vi "SquareFilter1.vi"(3 "error IN":errorcluster, 4 "Areas":dbl[][](array[numeric]), 5 "X,Y":dbl[][](array[numeric]), 6 "Chains (X,Y,dX,dY)":dbl[][](array[numeric])) -> (0 "error OUT":errorcluster, 1 "Finded False Displac":i32, 2 "Filtered Chains (X,Y,dX,dY)":dbl[][](array[numeric]))   [LabVIEW 2013]
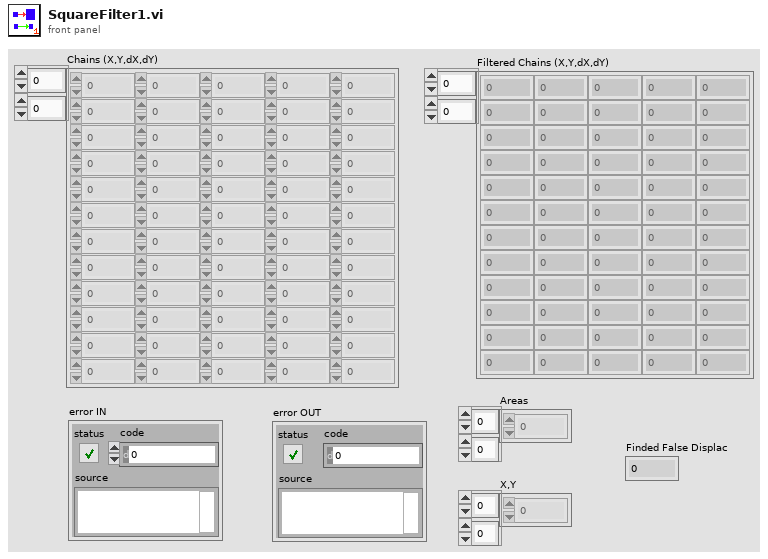
[diagram p1: front panel]
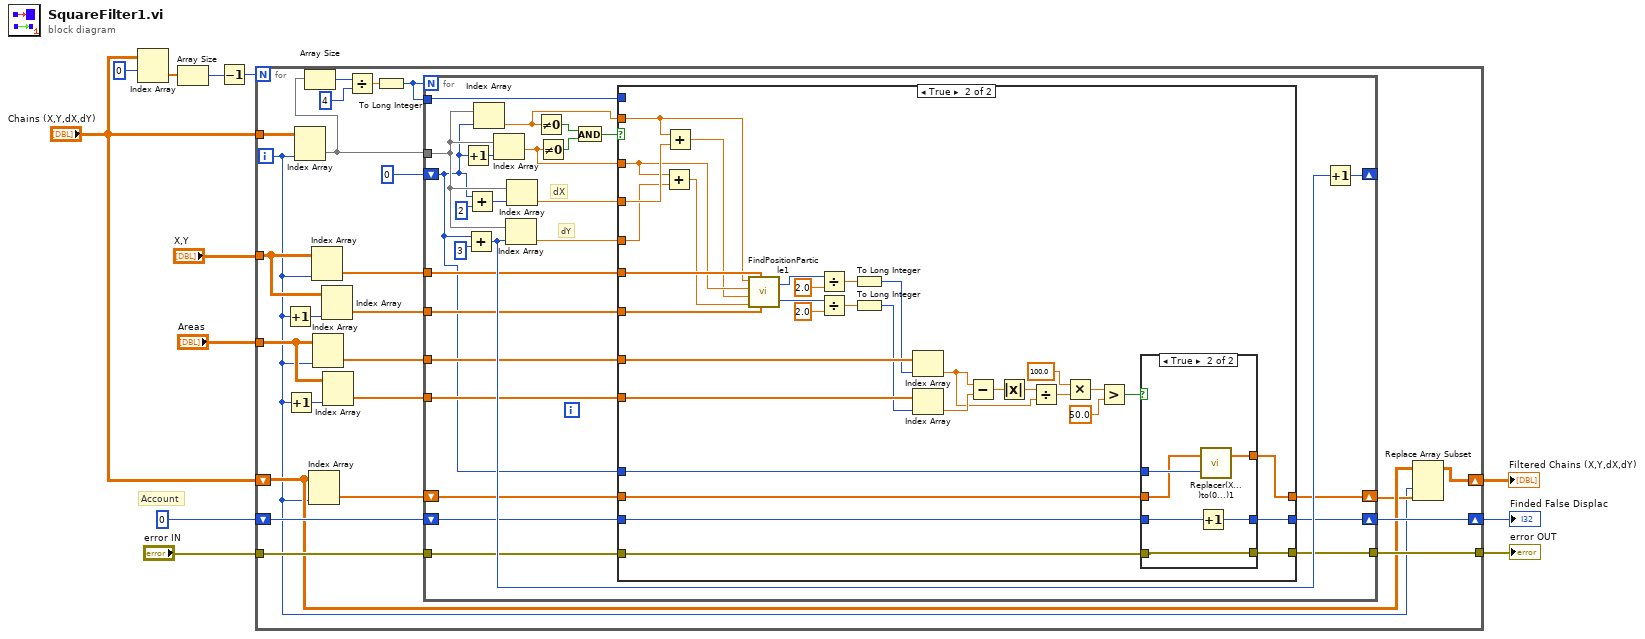
[diagram p0: block diagram]
diagram:
  # "Account"
  n1 = Index Array(array="Chains (X,Y,dX,dY)", index (row)=0) -> (element=w11:dbl[])  [unwired: 1 in]
  n2 = Array Size(array=w11) -> (size(s)=w4:i32)
  n3 = Decrement(x=w4) -> (x-1=w3:i32)
  n4 = for {
    N: w3 -> [_]
    tunnel: "error IN" -> [w33]
    tunnel: "Chains (X,Y,dX,dY)" -> [w31]
    shift-right: [w14] -> w6
    shift-left: "Chains (X,Y,dX,dY)" -> [w16]
    tunnel: [w30] -> w8
    shift-right: [w28] -> w7
    shift-left: 0 -> [w29]
    tunnel: "Areas" -> [w20]
    tunnel: "X,Y" -> [w25]
    i -> [w13]
    n5 = Increment(x=w13) -> (x+1=w24:i32)
    n6 = Increment(x=w13) -> (x+1=w21:i32)
    n7 = Index Array(array=w31, index (col)=w13) -> (element=w34:dbl[])  [unwired: 1 in]
    n8 = Array Size(array=w34) -> (size(s)=w36:i32)
    n9 = Index Array(array=w16, index (col)=w13) -> (element=w17:dbl[])  [unwired: 1 in]
    n10 = Index Array(array=w25, index (col)=w13) -> (element=w23:dbl[])  [unwired: 1 in]
    n11 = Index Array(array=w20, index (col)=w13) -> (element=w19:dbl[])  [unwired: 1 in]
    n12 = Index Array(array=w25, index (col)=w24) -> (element=w22:dbl[])  [unwired: 1 in]
    n13 = Index Array(array=w20, index (col)=w21) -> (element=w18:dbl[])  [unwired: 1 in]
    n14 = Divide(x=w36, y=4) -> (x/y=w27:dbl)
    n15 = To Long Integer(number=w27) -> (32bit integer=w26:i32)
    n16 = for {
      N: w26 -> [_]
      tunnel: w33 -> [w47]
      shift-right: [w53] -> _
      shift-left: 0 -> [w38]
      tunnel: w26 -> [w55]
      tunnel: w34 -> [w54]
      tunnel: [w46] -> w30
      shift-right: [w44] -> w28
      shift-left: w29 -> [w45]
      tunnel: w23 -> [w43]
      tunnel: w22 -> [w42]
      tunnel: w19 -> [w41]
      tunnel: w18 -> [w40]
      shift-right: [w37] -> w15
      shift-left: w17 -> [w39]
      # "dY"
      # "dX"
      n17 = Increment(x=w38) -> (x+1=w62:i32)
      n18 = Add(x=w38, y=3) -> (x+y=w52:i32)
      n19 = Add(x=w38, y=2) -> (x+y=w61:i32)
      n20 = Index Array(array=w54, index=w38) -> (element=w50:dbl)
      n21 = Index Array(array=w54, index=w62) -> (element=w51:dbl)
      n22 = Index Array(array=w54, index=w52) -> (element=w48:dbl)
      n23 = Index Array(array=w54, index=w61) -> (element=w49:dbl)
      n24 = Not Equal To 0?(x=w50) -> (x != 0?=w58:bool)
      n25 = Not Equal To 0?(x=w51) -> (x != 0?=w57:bool)
      n26 = And(x=w58, y=w57) -> (x .and. y?=w56:bool)
      n27 = case shown="True" w56 {
        tunnel: w55 -> [_ _]
        tunnel: w51 -> [_ w94]
        tunnel: w50 -> [_ w95]
        tunnel: w49 -> [_ w99]
        tunnel: w48 -> [_ w98]
        tunnel: [w65 w72] -> w46
        tunnel: w47 -> [w65 w71]
        tunnel: w45 -> [w64 w70]
        tunnel: [w64 w69] -> w44
        tunnel: w43 -> [_ w97]
        tunnel: w42 -> [_ w96]
        tunnel: w41 -> [_ w87]
        tunnel: w40 -> [_ w83]
        tunnel: w39 -> [w63 w68]
        tunnel: w38 -> [_ w67]
        tunnel: [w63 w66] -> w37
        frame False {
        }
        frame True {
          n28 = Add(x=w94, y=w98) -> (x+y=w92:dbl)
          n29 = Add(x=w95, y=w99) -> (x+y=w93:dbl)
          n30 = call "FindPositionParticle1.vi"("X,Y (2Frame)"=w96, "X,Y (1Frame)"=w97, "Y2"=w92, "X2"=w93, "Y1"=w94, "X1"=w95) -> ("Index X2"=w88:i32, "Index X1"=w90:i32)
          n31 = Divide(x=w90, y=2.0) -> (x/y=w86:dbl)
          n32 = Divide(x=w88, y=2.0) -> (x/y=w85:dbl)
          n33 = To Long Integer(number=w86) -> (32bit integer=w84:i32)
          n34 = To Long Integer(number=w85) -> (32bit integer=w82:i32)
          n35 = Index Array(array=w87, index=w84) -> (element=w78:dbl)
          n36 = Index Array(array=w83, index=w82) -> (element=w81:dbl)
          n37 = Subtract(x=w78, y=w81) -> (x-y=w80:dbl)
          n38 = Absolute Value(x=w80) -> (abs(x)=w79:dbl)
          n39 = Divide(x=w79, y=w78) -> (x/y=w77:dbl)
          n40 = Multiply(x=100.0, y=w77) -> (x*y=w75:dbl)
          n41 = Greater?(x=w75, y=50.0) -> (0:w73:bool)
          n42 = case shown="True" w73 {
            tunnel: [w100 w108] -> w72
            tunnel: w71 -> [w100 w108]
            tunnel: w70 -> [w102 w107]
            tunnel: [w102 w106] -> w69
            tunnel: w68 -> [w101 w104]
            tunnel: w67 -> [_ w105]
            tunnel: [w101 w103] -> w66
            frame False {
            }
            frame True {
              n43 = Increment(x=w107) -> (x+1=w106:i32)
              n44 = call "Replacer(X...)to(0...)1.vi"("Started index"=w105, "Arra in"=w104) -> ("Replaced array"=w103:dbl[])  [unwired: 1 out]
            }
          }
        }
      }
      n45 = Increment(x=w52) -> (x+1=w53:i32)
    }
    n46 = Replace Array Subset(array=w16, new element=w15, index (col)=w13) -> (w14:dbl[][])  [unwired: 1 in]
  }
  "error OUT" <- w8
  "Finded False Displac" <- w7
  "Filtered Chains (X,Y,dX,dY)" <- w6
